vi "Read Front Tunnel Internal TermRefs.vi"(8 "error in (no error)":errorcluster, 10 "case":string, 11 "CSM-Helper in":refnum<class "CSM-Helper.lvclass">) -> (0 "error out":errorcluster, 2 "Front Tunnels":T1, 3 "CSM-Helper out":refnum<class "CSM-Helper.lvclass">)   [LabVIEW 2017, in "CSM-Helper.lvclass"]
doc: "### Read Front Tunnel Internal TermRefs.vi\n\n-- <b>Controls</b> --\n- <b>case</b>:\n- <b>CSM-Helper in</b>: CSMHelper input\n\n-- <b>Indicators</b> --\n- <b>Front Tunnels</b>:\n- <b>CSM-Helper out</b>: CSMHelper output"
uses:
  CSM-Helper.lvclass
  CSM-Helper.lvclass/CSM-Helper.ctl
  Read Front Tunnels Refs.vi
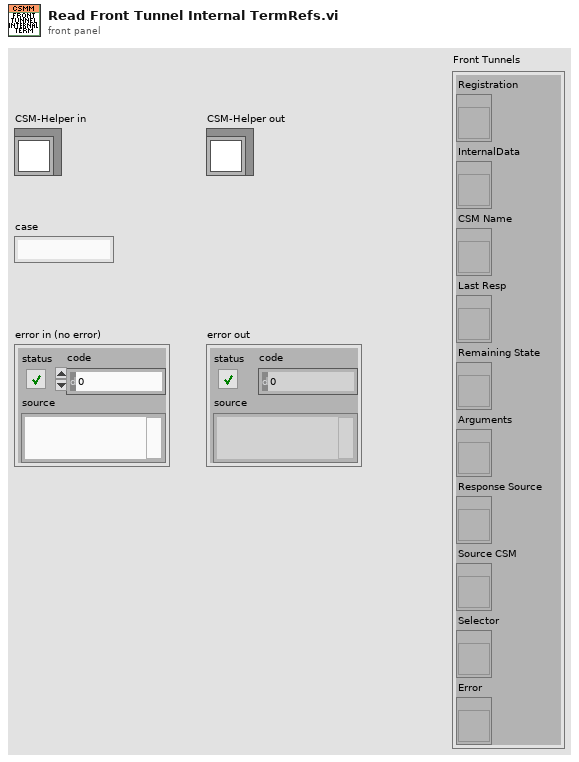
[diagram p1: front panel]
types:
  T1 = cluster{"Registration":refnum<vi>, "InternalData":refnum<vi>, "CSM Name":refnum<vi>, "Last Resp":refnum<vi>, "Remaining State":refnum<vi>, "Arguments":refnum<vi>, "Response Source":refnum<vi>, "Source CSM":refnum<vi>, "Selector":refnum<vi>, "Error":refnum<vi>}
  T2 = typedef "CSM-Helper.lvclass/_csmhelper_Front_Tunnels_Refs.ctl" = cluster{"Registration":refnum<vi>, "InternalData":refnum<vi>, "CSM Name":refnum<vi>, "Last Resp":refnum<vi>, "Remaining State":refnum<vi>, "Arguments":refnum<vi>, "Response Source":refnum<vi>, "Source CSM":refnum<vi>, "Selector":refnum<vi>, "Error":refnum<vi>}
  T3 = cluster{refnum<vi>, refnum<vi>, refnum<vi>, refnum<vi>, refnum<vi>, refnum<vi>, refnum<vi>, refnum<vi>, refnum<vi>, refnum<vi>}
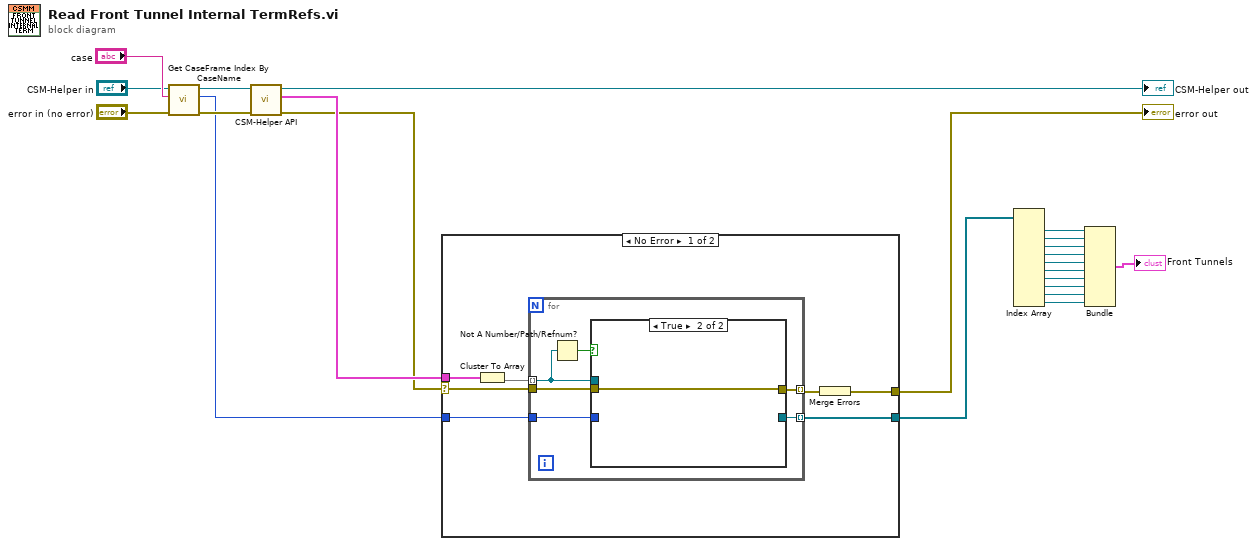
[diagram p0: block diagram]
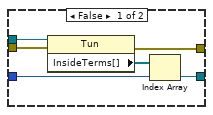
[diagram p2: hidden frame]
diagram:
  n1 = call "Get CaseFrame Index By CaseName.vi"("error in (no error)"="error in (no error)", "CASE"="case", "CSM-Helper in"="CSM-Helper in") -> ("error out"=w21:errorcluster, "index"=w15:i32, "CSM-Helper out"=w19:refnum<class "CSM-Helper.lvclass">)  [unwired: 5 in, 1 out]
  n2 = call-poly "CSM-Helper API.vi"("error in (no error)"=w21, "CSM-Helper in"=w19) -> ("error out"=w13:errorcluster, "Front Tunnels"=w22:T2, "CSM-Helper out"=→"CSM-Helper out":refnum<class "CSM-Helper.lvclass">)  [unwired: 7 in]
  n3 = case shown="No Error" w13 {
    selector: w13 -> [w24 w43]
    tunnel: w22 -> [w29 _]
    tunnel: w15 -> [w28 _]
    tunnel: [w27 _] -> w14
    tunnel: [w23 w43] -> w12
    frame No Error {
      n4 = Cluster To Array(cluster=w29) -> (array=w26:refnum<vi>[])
      n5 = for {
        tunnel: w28 -> [w35]
        tunnel: [w34] -> w27 mode=indexing
        tunnel: w26 -> [w31] mode=indexing
        tunnel: w24 -> [w33]
        tunnel: [w32] -> w25 mode=indexing
        n6 = Not A Number/Path/Refnum?(number/path/refnum=w31) -> (NaN/Path/Refnum?=w30:bool)
        n7 = case shown="True" w30 {
          tunnel: w35 -> [w40 _]
          tunnel: [w39 _] -> w34
          tunnel: w33 -> [w38 w42]
          tunnel: [w37 w42] -> w32
          tunnel: w31 -> [w36 _]
          frame False {
            n8 = property on="Property Node" class="Tun"(reference=w36, error in=w38) -> (error out=w37:errorcluster, "InsideTerms[]"=w41:refnum<vi>[])  [unwired: 1 out]
            n9 = Index Array(array=w41, index=w40) -> (element=w39:refnum<vi>)
          }
          frame True {
          }
        }
      }
      n10 = Merge Errors(w25) -> (w23:errorcluster)
    }
    frame Error {
    }
  }
  "error out" <- w12
  n11 = Index Array(array=w14) -> (element #1=w11:refnum<vi>, element #2=w10:refnum<vi>, element #3=w9:refnum<vi>, element #4=w8:refnum<vi>, element #5=w7:refnum<vi>, element #6=w6:refnum<vi>, element #7=w5:refnum<vi>, element #8=w4:refnum<vi>, element #9=w3:refnum<vi>, element #10=w1:refnum<vi>)  [unwired: 10 in]
  n12 = Bundle(w11, w10, w9, w8, w7, w6, w5, w4, w3, w1) -> (→"Front Tunnels":T3)  [unwired: 1 in]
